vi "Export.vi"(8 "error in":errorcluster, 10 "path":path, 11 "item in":T1 format="%.0x") -> (0 "error out":errorcluster, 3 "item out":T1 format="%.0x")   [LabVIEW 2017, in "Import Export.lvlib"]
uses:
  <vilib>/NI Veristand/Custom Device API/Custom Device Item Ref.ctl
  NationalInstruments.VeriStand.SystemDefinitionAPI
  NationalInstruments.VeriStand.SystemStorage
  Import Export.lvlib
  <vilib>/NI Veristand/Custom Device API/Custom Device API.lvlib
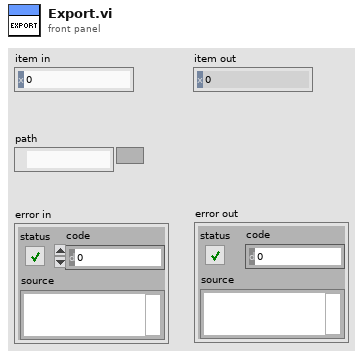
[diagram p1: front panel]
types:
  T1 = typedef "Custom Device API.lvlib/Custom Device Item Ref.ctl" = u64
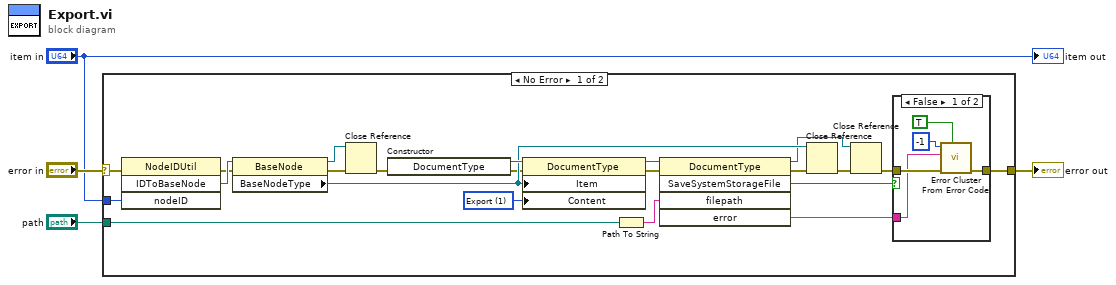
[diagram p0: block diagram]
diagram:
  n1 = case shown="No Error" "error in" {
    selector: "error in" -> [w22 w33]
    tunnel: "path" -> [w17 _]
    tunnel: [w9 w33] -> w2
    tunnel: "item in" -> [w21 _]
    frame No Error {
      w5 = 1 items=["Definition", "Export", "SLSC"] ("Content")
      n2 = invoke class="NodeIDUtil" method="IDToBaseNode"(error in=w22, "nodeID"=w21) -> (error out=w20:errorcluster, "IDToBaseNode"=w23:refnum<k24>)  [unwired: 2 in, 2 out]
      n3 = property class="BaseNode"(reference=w23, error in=w20) -> (reference out=w18:refnum<k24>, error out=w19:errorcluster, "BaseNodeType"=w16:refnum<k24>)
      n4 = Close Reference(reference=w18, error in (no error)=w19) -> (error out=w15:errorcluster)
      n5 = constructor class="DocumentType"(error in=w15) -> (reference out=w24:refnum<k24>, error out=w14:errorcluster)  [unwired: 2 in, 1 out]
      n6 = property class="DocumentType"(reference=w24, error in=w14, "Item"=w16, "Content"=w5) -> (reference out=w25:refnum<k24>, error out=w8:errorcluster)
      n7 = Path To String(path=w17) -> (string=w26:string)
      n8 = invoke class="DocumentType" method="SaveSystemStorageFile"(reference=w25, error in=w8, "filepath"=w26) -> (reference out=w13:refnum<k24>, error out=w7:errorcluster, "SaveSystemStorageFile"=w12:bool, "error"=w11:string)  [unwired: 2 in, 1 out]
      n9 = Close Reference(reference=w16, error in (no error)=w7) -> (error out=w6:errorcluster)
      n10 = Close Reference(reference=w13, error in (no error)=w6) -> (error out=w10:errorcluster)
      n11 = case shown="False" w12 {
        tunnel: [w29 w32] -> w9
        tunnel: w10 -> [w30 w32]
        tunnel: w11 -> [w27 _]
        frame False {
          n12 = call <vilib>:"Error Cluster From Error Code.vi"("show call chain? (False)"=TRUE, "error in (no error)"=w30, "error message (\"\")"=w27, "error code (0)"=-1) -> ("error out"=w29:errorcluster)  [unwired: 5 in]
        }
        frame True {
        }
      }
    }
    frame Error {
    }
  }
  "error out" <- w2
  "item out" <- "item in"
